vi "Teleop.vi"(10 "Match Info":T2={"Autonomous Elapsed Seconds"=0.0, "TeleOp Elapsed Seconds"=0.0, "Disabled Elapsed Seconds"=0.0, "Visited Autonomous"=FALSE, "Visited TeleOp"=FALSE, "Visited Disabled"=FALSE, "Autonomous Settings"={"Autonomous Style"=enum."Independent", "VI Refnum"=refnum}}, 11 "Call Context":T3) -> ()   [LabVIEW 2020]
doc: "This VI is called for each TeleOp packet received from the DS where the robot is not disabled. It is often used to read from the joysticks and update I/O or to update setpoints for timed control loops. It should complete and return within 20 milliseconds or it may miss DS packets."
uses:
  <vilib>/Rock Robotics/WPI/DriverStation/WPI_DriverStationDerivedRobotMode.ctl
  <vilib>/Rock Robotics/WPI/DriverStation/WPI_DriverStationMatch Info.ctl
  <vilib>/Rock Robotics/WPI/ThirdParty/Phoenix-LabVIEW/Motor Controller/Controls/CTRE_Phoenix_MotorControl_ControlMode.ctl
  <vilib>/Rock Robotics/WPI/Utilities/WPI_GetSetVariantRefNum.vi
  <vilib>/Rock Robotics/WPI/ThirdParty/Phoenix-LabVIEW/Motor Controller/Get/CTRE_Phoenix_MotorController_GetSupplyAndStatorCurrent_Enhanced.vi
  TitanLib/Lib/TitanLib.lvlib
  <vilib>/Rock Robotics/Network Tables/NT Write Boolean Array.vi
  <vilib>/Rock Robotics/Network Tables/NT Write Numeric Array.vi
  TitanLib/Lib/RPMToRawUnits-2048-CPR.vi
  <vilib>/Rock Robotics/WPI/ThirdParty/Phoenix-LabVIEW/Motor Controller/Get/CTRE_Phoenix_MotorController_GetSelectedSensorData.vi
  TitanLib/Lib/RawUnitsToRPM-2048-CPR.vi
panel:
  in  "I Zone":dbl=1000.0
  out "Raw Units":i32
  in  "F":dbl=0.0461
  in  "D":dbl
  in  "I":dbl=0.001
  in  "P":dbl=0.1
  in  "Set PIDF":bool=TRUE
  in  "Setpoint RPM":dbl=7000.0
  out "Shooter Motor Current":T1(graph)
  out "Rpm":dbl(graph)
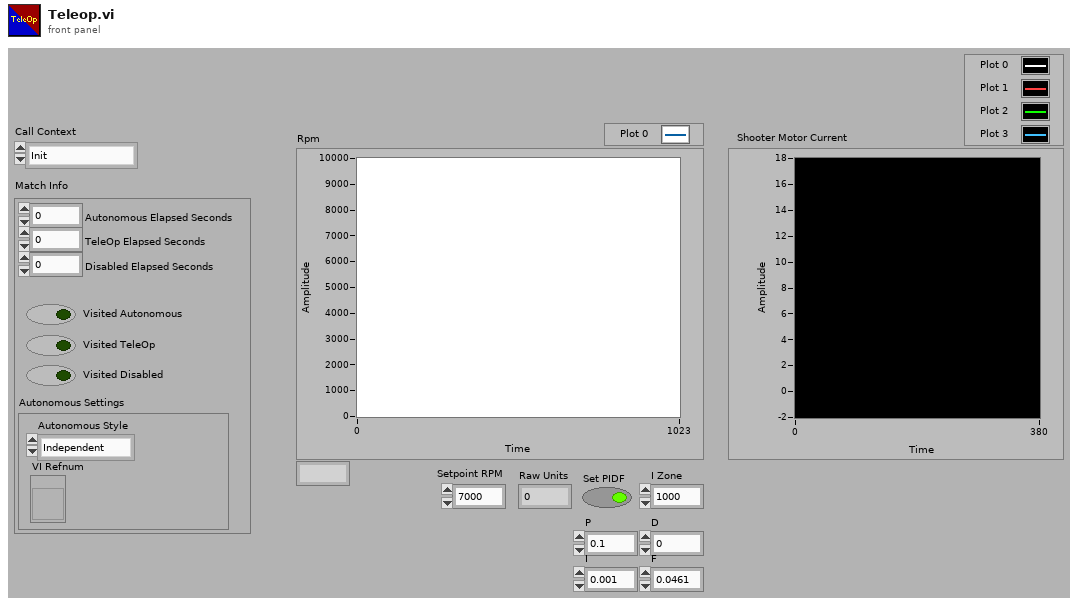
[diagram p1: front panel]
types:
  T1 = cluster{"Supply Current":dbl, "Stator Current":dbl, "Supply Current":dbl, "Stator Current":dbl}
  T2 = typedef "WPI_DriverStationMatch Info.ctl" = cluster{"Autonomous Elapsed Seconds":dbl, "TeleOp Elapsed Seconds":dbl, "Disabled Elapsed Seconds":dbl, "Visited Autonomous":bool, "Visited TeleOp":bool, "Visited Disabled":bool, "Autonomous Settings":cluster{"Autonomous Style":enum16{"Iterative", "Independent"}, "VI Refnum":refnum<vi>}}
  T3 = typedef "WPI_DriverStationDerivedRobotMode.ctl" = enum16{"Init", "Execute", "Stop"}
  T4 = typedef "CTRE_Phoenix_MotorControl_ControlMode.ctl" = u16
  T5 = typedef "WPI_JoystickDevRef.ctl" = cluster{"Device":T6}
  T6 = typedef "WPI_JoystickDeviceEnum.ctl" = enum16{"USB 0", "USB 1", "USB 2", "USB 3", "USB 4", "USB 5"}
  T7 = typedef "WPI_MotorControlDeviceRef.ctl" = cluster{"DeviceStatus":errorcluster, "Type":T8, "PWM":cluster{"PWM Channel":T9, "DeadBand":T10}, "CAN":cluster{"Device Number":u8, "SetOutput VI Ref":variant, "GetOutput VI Ref":variant, "Enable VI Ref":variant, "Disable VI Ref":variant, "Data":variant}, "Invert":bool, "DIO PWM":cluster{"PWM \"Enable\" Channel":T9, "DIOChannel":T11, "PWM Rate":dbl}}
  T8 = typedef "WPI_MotorControlType.ctl" = enum16{"PWM", "CAN", "DIO PWM"}
  T9 = typedef "FPGA_DIOPWMChannel.ctl" = enum8{"PWM 0", "PWM 1", "PWM 2", "PWM 3", "PWM 4", "PWM 5", "PWM 6", "PWM 7", "PWM 8", "PWM 9", "PWM MXP 0", "PWM MXP 1", "PWM MXP 2", "PWM MXP 3", "PWM MXP 4", "PWM MXP 5", "PWM MXP 6", "PWM MXP 7", "PWM MXP 8", "PWM MXP 9", "Invalid"}
  T10 = typedef "WPI_PWMDeadband.ctl" = cluster{"Name":string, "maxPositivePwm":i32, "minPositivePwm":i32, "centerPwm":i32, "maxNegativePwm":i32, "minNegativePwm":i32, "angularRange":u16}
  T11 = typedef "FPGA_DIOChannel.ctl" = enum8{"DIO 0", "DIO 1", "DIO 2", "DIO 3", "DIO 4", "DIO 5", "DIO 6", "DIO 7", "DIO 8", "DIO 9", "DIO MXP 0", "DIO MXP 1", "DIO MXP 2", "DIO MXP 3", "DIO MXP 4", "DIO MXP 5", "DIO MXP 6", "DIO MXP 7", "DIO MXP 8", "DIO MXP 9", "DIO MXP 10", "DIO MXP 11", "DIO MXP 12", "DIO MXP 13", "DIO MXP 14", "DIO MXP 15", "SPI Port CS1", "SPI Port CS2", "SPI Port CS3", "SPI Port MISO", "SPI Port MOSI", "Invalid"}
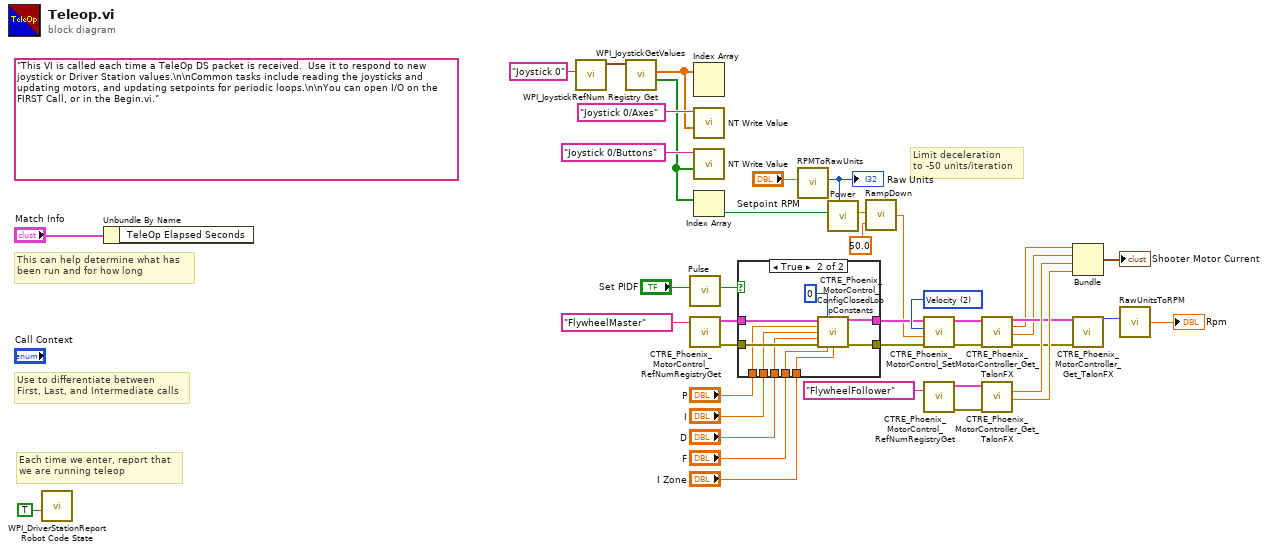
[diagram p0: block diagram]
diagram:
  w32 = T4 2 items=["PercentOutput"=0, "Position"=1, "Velocity"=2, "Current"=3, "Follower"=5, "MotionProfile"=6, "MotionMagic"=7, "MotionProfileArc"=10, "Disabled"=15] ("Control Mode")
  (unwired) "This VI is called each time a TeleOp DS packet is received.  Use it to respond to new joystick or Driver Station values.\n\nCommon tasks include reading the joysticks and updating motors, and updating setpoints for periodic loops.\n\nYou can open I/O on the FIRST Call, or in the Begin.vi."
  # "Limit deceleration\nto -50 units/iteration"
  # "Each time we enter, report that\nwe are running teleop"
  # "Use to differentiate between\nFirst, Last, and Intermediate calls"
  # "This can help determine what has\nbeen run and for how long"
  n1 = call <vilib>:"WPI_DriverStationReport Robot Code State.vi"("TeleOp"=TRUE ("Autonomous")) -> ()  [unwired: 10 in, 1 out]
  n2 = Unbundle By Name("Match Info") -> ()  [unwired: 1 out]
  n3 = call <vilib>:"WPI_JoystickRefNum Registry Get.vi"("refnum name"="Joystick 0") -> ("JoystickDevRef"=w39:T5)  [unwired: 1 in, 9 out]
  n4 = call <vilib>:"WPI_JoystickGetValues.vi"("JoystickDevRef"=w39) -> ("Buttons"=w4:bool[], "Axes"=w35:dbl[])  [unwired: 6 in, 3 out]
  n5 = call "Pulse.vi"("Input"="Set PIDF") -> ("Output"=w22:bool)  [unwired: 10 in]
  n6 = call <vilib>:"CTRE_Phoenix_MotorControl_RefNumRegistryGet.vi"("refnum name"="FlywheelMaster") -> ("error out"=w24:errorcluster, "PhoenixMotorControlDevRef"=w25:T7)  [unwired: 9 in]
  n7 = Index Array(array=w35) -> ()  [unwired: 2 in, 2 out]
  n8 = call-poly <vilib>:"NT Write Value.vi"("Numeric Array"=w35, "Name"="Joystick 0/Axes") -> ()  [unwired: 9 in, 1 out]
  n9 = call-poly <vilib>:"NT Write Value.vi"("Boolean Array"=w4, "Name"="Joystick 0/Buttons") -> ()  [unwired: 9 in, 1 out]
  n10 = Index Array(array=w4) -> (element=w5:bool)  [unwired: 1 in]
  n11 = case shown="True" w22 {
    tunnel: w25 -> [w43 w53]
    tunnel: w24 -> [w42 w52]
    tunnel: "P" -> [_ w51]
    tunnel: "I" -> [_ w50]
    tunnel: "D" -> [_ w49]
    tunnel: "F" -> [_ w48]
    tunnel: [w43 w46] -> w13
    tunnel: [w42 w45] -> w12
    tunnel: "I Zone" -> [_ w44]
    frame False {
    }
    frame True {
      n12 = call <vilib>:"CTRE_Phoenix_MotorControl_ConfigClosedLoopConstants.vi"("PhoenixMotorControlDevRef"=w53, "slotIdx"=0, "P"=w51, "I"=w50, "D"=w49, "error in (no error)"=w52, "F"=w48, "I Zone"=w44) -> ("PhoenixMotorControlDevRef"=w46:T7, "error out"=w45:errorcluster)  [unwired: 6 in]
    }
  }
  n13 = call-poly "RPMToRawUnits.vi"("RPM"="Setpoint RPM") -> ("Raw Units"=w8:i32)  [unwired: 3 in]
  "Raw Units" <- w8
  n14 = call "Power.vi"("Positive Power"=w8, "Positive"=w5) -> ("Output"=w3:dbl)  [unwired: 9 in]
  n15 = call "RampDown.vi"("Decrease per Cycle"=50.0, "Input"=w3) -> ("Output"=w2:dbl)
  n16 = call <vilib>:"CTRE_Phoenix_MotorControl_Set.vi"("error in (no error)"=w12, "Output"=w2, "Control Mode"=w32, "PhoenixMotorControlDevRef"=w13) -> ("error out"=w15:errorcluster, "PhoenixMotorControlDevRef"=w16:T7)  [unwired: 6 in]
  n17 = call <vilib>:"CTRE_Phoenix_MotorControl_RefNumRegistryGet.vi"("refnum name"="FlywheelFollower") -> ("error out"=w10:errorcluster, "PhoenixMotorControlDevRef"=w11:T7)  [unwired: 9 in]
  n18 = call-poly <vilib>:"CTRE_Phoenix_MotorController_Get_TalonFX.vi"("PhoenixMotorControlDevRef"=w16, "error in"=w15) -> ("PhoenixMotorControlDevRef"=w29:T7, "Supply Current"=w27:dbl, "Stator Current"=w26:dbl, "error out"=w28:errorcluster)  [unwired: 10 in]
  n19 = call-poly <vilib>:"CTRE_Phoenix_MotorController_Get_TalonFX.vi"("PhoenixMotorControlDevRef"=w11, "error in"=w10) -> ("Supply Current"=w31:dbl, "Stator Current"=w30:dbl)  [unwired: 10 in, 2 out]
  n20 = Bundle("Supply Current"=w27, "Stator Current"=w26, "Supply Current"=w31, "Stator Current"=w30) -> (→"Shooter Motor Current":T1)  [unwired: 1 in]
  n21 = call-poly <vilib>:"CTRE_Phoenix_MotorController_Get_TalonFX.vi"("PhoenixMotorControlDevRef"=w29, "error in"=w28) -> ("Velocity (Raw Sensor Units per 100 ms)"=w7:i32)  [unwired: 10 in, 3 out]
  n22 = call-poly "RawUnitsToRPM.vi"("Raw Units"=w7) -> ("RPM"=→"Rpm":dbl)  [unwired: 3 in]
